vi "Get Refnum From Label.vi"(7 "label":string, 8 "label array in":string[](array[string]), 11 "controls[] in":refnum<vi>[](array[refnum])) -> (0 "label array out":string[](array[string]), 3 "controls[] out":refnum<vi>[](array[refnum]), 4 "refnum out":refnum<vi>)   [LabVIEW 2018]
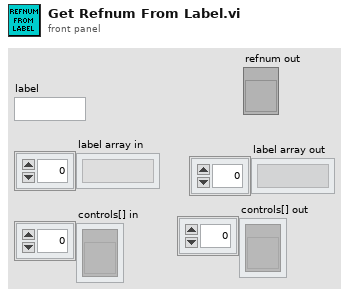
[diagram p1: front panel]
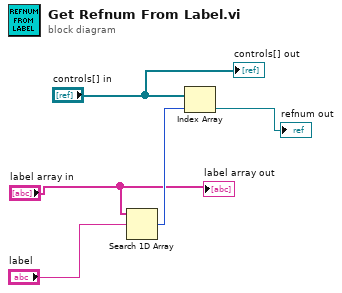
[diagram p0: block diagram]
diagram:
  n1 = Search 1D Array(1D array="label array in", element="label") -> (index of element=w5:i32)  [unwired: 1 in]
  n2 = Index Array(array="controls[] in", index=w5) -> (element=→"refnum out":refnum<vi>)
  "controls[] out" <- "controls[] in"
  "label array out" <- "label array in"
